vi "Get Sinlgeton.vi"(11 "Singleton in":refnum<class "Singleton.lvclass">) -> (3 "Singleton out":refnum<class "Singleton.lvclass">)   [LabVIEW 2020, in "Singleton.lvclass"]
uses:
  Singleton.lvclass
  Singleton.lvclass/Singleton.ctl
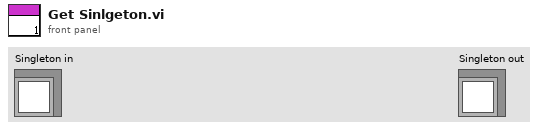
[diagram p1: front panel]
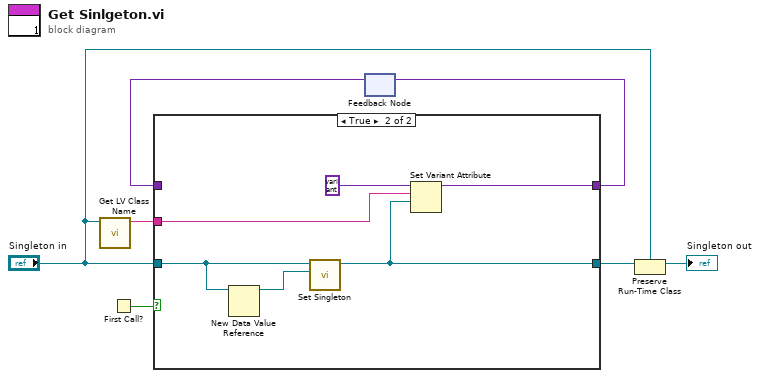
[diagram p0: block diagram]
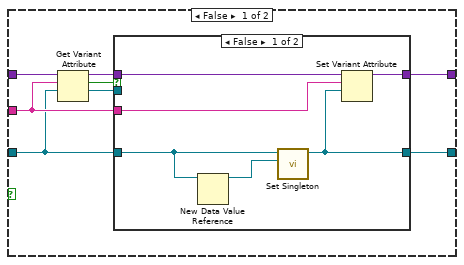
[diagram p2: hidden frame]
diagram:
  n1 = call <vilib>:"Get LV Class Name.vi"("object"="Singleton in") -> ("class name"=w6:string)  [unwired: 9 in, 1 out]
  n2 = First Call?() -> (First Call?: T/F=w7:bool)
  n3 = feedback #1() -> (w4:variant)  [unwired: 1 in]
  n4 = case shown="True" w7 {
    tunnel: "Singleton in" -> [w8 w29]
    tunnel: w6 -> [w12 w26]
    tunnel: [w11 w25] -> w5
    tunnel: w4 -> [w15 _]
    tunnel: [w10 w24] -> w3
    frame False {
      n5 = Get Variant Attribute(Variant=w15, name=w12, default value (empty Variant)=w8) -> (duplicate Variant=w14:variant, found=w13:bool, value=w9:refnum<class "Singleton.lvclass">)  [unwired: 1 in, 1 out]
      n6 = case shown="False" w13 {
        tunnel: w14 -> [w19 w23]
        tunnel: w8 -> [w20 _]
        tunnel: w12 -> [w18 _]
        tunnel: [w17 w23] -> w11
        tunnel: [w16 w22] -> w10
        tunnel: w9 -> [_ w22]
        frame False {
          n7 = New Data Value Reference(data value=w20) -> (data value reference=w21:refnum<data-value>)  [unwired: 1 in, 1 out]
          n8 = call "Set Singleton.vi"("singleton"=w21, "Singleton in"=w20) -> ("Singleton out"=w16:refnum<class "Singleton.lvclass">)  [unwired: 8 in, 1 out]
          n9 = Set Variant Attribute(Variant=w19, name=w18, value=w16) -> (Variant out=w17:variant)  [unwired: 1 in, 2 out]
        }
        frame True {
        }
      }
    }
    frame True {
      n10 = New Data Value Reference(data value=w29) -> (data value reference=w28:refnum<data-value>)  [unwired: 1 in, 1 out]
      n11 = call "Set Singleton.vi"("singleton"=w28, "Singleton in"=w29) -> ("Singleton out"=w24:refnum<class "Singleton.lvclass">)  [unwired: 8 in, 1 out]
      n12 = Set Variant Attribute(Variant=variant, name=w26, value=w24) -> (Variant out=w25:variant)  [unwired: 1 in, 2 out]
    }
  }
  n13 = feedback-in #1(w5) -> ()
  n14 = Preserve Run-Time Class(object in=w3, 2:"Singleton in") -> (object out=→"Singleton out":refnum<class "Singleton.lvclass">)  [unwired: 1 in, 1 out]
